vi "isInBound.vi"(8 "error in (no error)":errorcluster, 10 "XY":cluster{"X":dbl, "Y":dbl}, 11 "QControl_Graph in":refnum<class "QControl_Graph.lvclass">) -> (0 "error out":errorcluster, 2 "Boolean":bool, 3 "QControl_Graph out":refnum<class "QControl_Graph.lvclass">)   [LabVIEW 2017, in "QControl_Graph.lvclass"]
uses:
  QControl_Graph.lvclass
  C:/Program Files (x86)/National Instruments/LabVIEW 2017/vi.lib/QSI/QControls/QControl Classes/GraphChart/GraphChart.lvclass
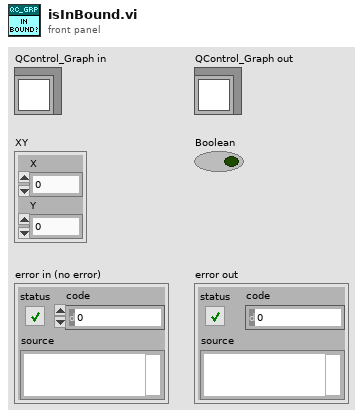
[diagram p1: front panel]
types:
  T1 = typedef "LVRectTypeDef.ctl" = cluster{"Left":i16, "Top":i16, "Right":i16, "Bottom":i16}
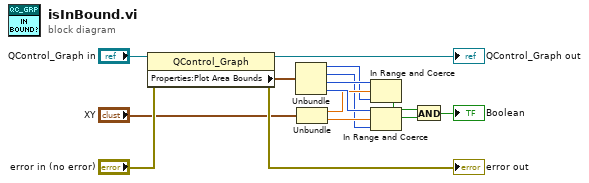
[diagram p0: block diagram]
diagram:
  n1 = property on="Property Node" class="QControl_Graph"(reference="QControl_Graph in", error in="error in (no error)") -> (reference out=→"QControl_Graph out":refnum<class "QControl_Graph.lvclass">, error out=→"error out":errorcluster, "Properties:Plot Area Bounds"=w9:T1)
  n2 = Unbundle(w9) -> ("Left"=w1:i16, "Top"=w2:i16, "Right"=w5:i16, "Bottom"=w6:i16)
  n3 = Unbundle("XY") -> ("X"=w4:dbl, "Y"=w3:dbl)
  n4 = In Range and Coerce(upper limit=w5, x=w4, lower limit=w1) -> (In Range?=w7:bool)  [unwired: 1 out]
  n5 = In Range and Coerce(upper limit=w6, x=w3, lower limit=w2) -> (In Range?=w8:bool)  [unwired: 1 out]
  n6 = And(x=w7, y=w8) -> (x .and. y?=→"Boolean":bool)
